vi "Get Engine.vi"(8 "error in (no error)":errorcluster, 11 "TSnax UI Manager in":refnum<class "TSnax UI Manager.lvclass">) -> (0 "error out":errorcluster, 2 "TSnax:Engine":refnum<class "Engine.lvclass">, 3 "TSnax UI Manager out":refnum<class "TSnax UI Manager.lvclass">)   [LabVIEW 2020, in "TSnax UI.lvlib" / "TSnax UI Manager.lvclass"]
uses:
  TSnax UI Manager.lvclass
  TSnax UI Manager.lvclass/TSnax UI Manager.ctl
  TSnax/Engine/Engine.lvclass
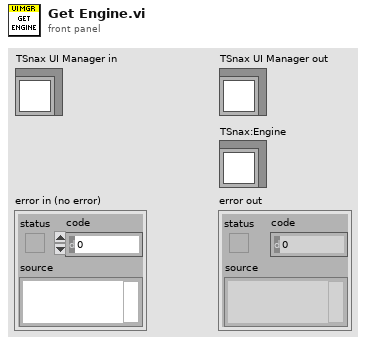
[diagram p1: front panel]
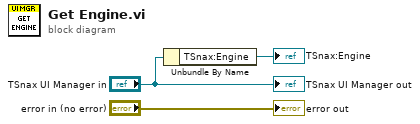
[diagram p0: block diagram]
diagram:
  n1 = Unbundle By Name("TSnax UI Manager in") -> ("TSnax:Engine"=→"TSnax:Engine":refnum<class "Engine.lvclass">)
  "error out" <- "error in (no error)"
  "TSnax UI Manager out" <- "TSnax UI Manager in"
